vi "Create.vi"(8 "error in (no error)":errorcluster, 9 "Calculation Period (ms)":u32=500, 10 "XNET Session":refnum<k21>, 11 "GenBus_Load_Calculator in":refnum<class "GenBus_Load_Calculator.lvclass">) -> (0 "error out":errorcluster, 3 "GenBus_Load_Calculator out":refnum<class "GenBus_Load_Calculator.lvclass">)   [LabVIEW 2019, in "XNET-Bus-Load-Calculator.lvlib" / "GenBus_Load_Calculator.lvclass"]
uses:
  GenBus_Load_Calculator.lvclass
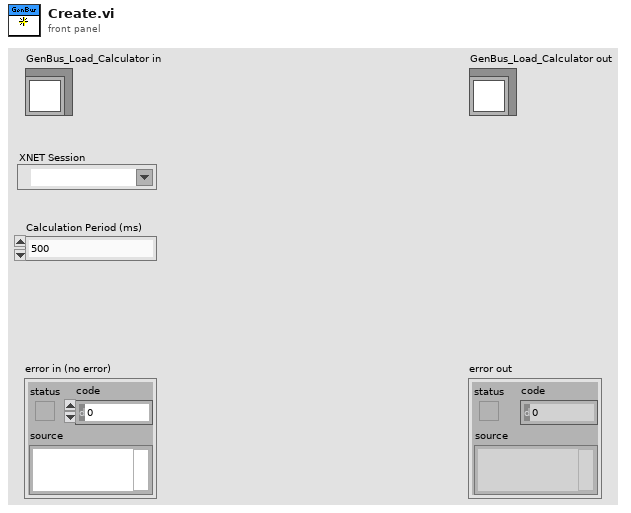
[diagram p1: front panel]
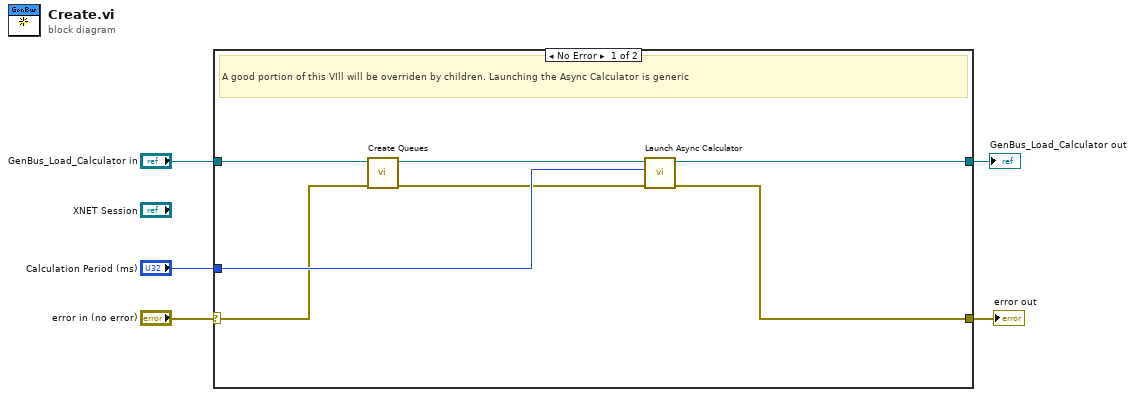
[diagram p0: block diagram]
diagram:
  n1 = case shown="No Error" "error in (no error)" {
    selector: "error in (no error)" -> [w7 w14]
    tunnel: [w10 w14] -> w4
    tunnel: [w12 w13] -> w2
    tunnel: "GenBus_Load_Calculator in" -> [w9 w13]
    tunnel: "Calculation Period (ms)" -> [w11 _]
    frame No Error {
      # "A good portion of this VIll will be overriden by children. Launching the Async Calculator is generic"
      n2 = call "Create Queues.vi"("error in (no error)"=w7, "GenBus_Load_Calculator in"=w9) -> ("error out"=w6:errorcluster, "GenBus_Load_Calculator out"=w8:refnum<class "GenBus_Load_Calculator.lvclass">)  [unwired: 8 in]
      n3 = call "Launch Async Calculator.vi"("error in (no error)"=w6, "Calculation Period (ms)"=w11, "Load Calculator in"=w8) -> ("error out"=w10:errorcluster, "Load Calculator out"=w12:refnum<class "GenBus_Load_Calculator.lvclass">)  [unwired: 7 in]
    }
    frame Error {
    }
  }
  "error out" <- w4
  "GenBus_Load_Calculator out" <- w2
